vi "McP Calibrate.vi"(0 "File Info In":T2={"FilePath"=path "/DATA/Labview Items", "Field (T)"=12.0, "Temperature (K)"=12.0, "X-Axis"=enum."nm", "Center nm"=-1.0, "Current Grating Density"=enum."600", "CCD Parameters"={"Exposure Time (s)"=0.2, "Offset"=0.0, "BkgrdCrct"=FALSE, "Shutter"=FALSE, "Mode"=enum."Regular", "Repetition"=4, "dt or s"=0.0}, "Operation Mode"=enum."NML Data Acquisition", "Exp Index"=3, "Index_repetition"=0, "Index"=0, "Current Detector"=enum."CCD-1024x256"} {"CCD Parameters"."dt or s" format="%#.6f"; "CCD Parameters"."Repetition" min=1; "CCD Parameters"."Offset" format="%#.2f"; "CCD Parameters"."Exposure Time (s)" min=0.02 max=6000.0 format="%#.2f"; "Center nm" format="%.2f"; "Temperature (K)" format="%.2f"; "Field (T)" format="%.2f"}, 11 "error in":errorcluster) -> (15 "error out":errorcluster)   [LabVIEW 2024]
doc: "If you enter this program by mistake, click RETURN to quit.\n\nCALIBRATION STEPS:\n\n(0) Make sure you have calibration source (Ne lamp, Hg lamp, etc.) set up correctly.\n(1) Select a calibration line.\n(2) Click Calibrate.\n The spectrometer will move to the selected calibration line wavelength, take a CCD shot and fit the result.\n(3)Check the calibration result. You will be prompt whether to accept the result.\n (3a)Click \"Cancel\" to leave the system unaltered.\n (3b)If you click \"OK\", the counter position will be set to the calibrated value.\nThe spectrometer will return to the original internal (stepper) position afterward."
uses:
  Globals and TypeDefs/Type Definitions.llb/FileInfoParameter.ctt
  Globals and TypeDefs/Type Definitions.llb/Wavelength Unit.ctt
  Globals and TypeDefs/Type Definitions.llb/McPherson Grating Density.ctl
  Globals and TypeDefs/Type Definitions.llb/CCDParameter.ctt
  Globals and TypeDefs/Type Definitions.llb/OperationMode.ctt
  Globals and TypeDefs/Type Definitions.llb/ListOfDetectors.ctt
  MCP/Calibration/GlobalCalLampInfo.vi
  Globals and TypeDefs/gSpectrometer.vi
  File and save/X-Axis_Generator_morph.vi
panel:
  in  "Rejecting":bool
  in  "Accepting":bool
  out "Standard Wavelengths":cluster{"Y":dbl[], "Y":dbl[]}[](graph)=[{"Y"=[302.70159912109375, 302.88641357421875, 319.8586120605469, 332.37451171875, 337.82159423828125, 352.047119140625, 376.6258850097656, 377.7132873535156, 540.05615234375, 585.248779296875, 602.9996948242188, 607.4337768554688, 614.3062744140625, 616.359375, 621.7281494140625, 626.6494750976562, 638.2991943359375, 640.2247924804688, 650.65283203125, 659.895263671875, 692.9467163085938, 703.2413330078125, 717.393798828125, 724.5166625976562, 837.7608032226562, 865.4382934570312, 878.062255859375, 878.3753051757812, 1114.302001953125, 1117.75244140625, 1152.2745361328125], "Y"=[300.0, 300.0, 500.0, 1000.0, 500.0, 100.0, 800.0, 1000.0, 200.0, 200.0, 100.0, 100.0, 100.0, 100.0, 100.0, 100.0, 100.0, 200.0, 150.0, 100.0, 1000.0, 800.0, 800.0, 800.0, 800.0, 600.0, 600.0, 400.0, 300.0, 500.0, 300.0]}, {"Y"=[205.28280639648438, 226.22230529785156, 253.65170288085938, 284.7674865722656, 296.7279968261719, 365.0152893066406, 398.3930969238281, 404.65631103515625, 435.8327941894531, 542.5253295898438, 546.073486328125, 567.7105102539062, 614.947509765625, 794.4555053710938, 1013.9760131835938], "Y"=[400.0, 400.0, 1000.0, 400.0, 250.0, 600.0, 1000.0, 400.0, 1000.0, 80.0, 500.0, 200.0, 250.0, 250.0, 200.0]}, {"Y"=[427.7528076171875, 434.806396484375, 460.9566955566406, 472.6867980957031, 476.48651123046875, 480.60198974609375, 487.98638916015625, 696.5430908203125, 706.7218017578125, 750.3869018554688, 763.5106201171875, 794.817626953125, 800.61572265625, 801.4785766601562, 810.3693237304688, 811.5311279296875, 912.2966918945312, 965.7786254882812], "Y"=[200.0, 250.0, 200.0, 200.0, 250.0, 200.0, 250.0, 300.0, 300.0, 600.0, 700.0, 600.0, 600.0, 700.0, 600.0, 1000.0, 1000.0, 700.0]}]
  in  "Range":T1={"X_Min"=0.3, "X_Max"=0.3, "Y_Min"=0.3, "Y-Max"=0.3}
  out "Solved Central WL":dbl=517.6607981427933 format="%.4f"
  in  "Searching center":dbl format="%.2f"
  in  "Recalculate":bool
  out "Pre-Cal WL":dbl=6000.0 min=0.0 max=26000.0 format="%.2f"
  out "Calibration State":T8(ring)
  in  "Return?":bool
  out "cursor position":dbl format="%.4f"
  in  "Points Between":i32=10 min=0 step=1
  out "Difference (cm-1)":dbl caption="(cm-1)" format="%#_3g"
  out "Difference (meV)":dbl caption="(meV)" format="%#_3g"
  out "Difference":dbl caption="(nm)" format="%#_3g"
  out "Calibrated Wavelenth(nm)":dbl=1000.0 format="%.4f"
  out "peak plot (post-cal":cluster{"X-axis":dbl[], dbl[]}[](graph)
  out "Full Data Plot":cluster{"X-axis":dbl[], "The Data":dbl[]}(graph)
  in  "Exposuretime (s)":dbl=0.5 format="%.2f"
  out "Pre & Current WL":dbl=692.9467 caption="PreCalibrated Wavelength (nm)" format="%.4f"
  in  "Select WL":u16(ring)=5 caption="Select a Calibration Line" items=["808.2458  nm  ( Ne )", "794.3181  nm  ( Ne )", "743.8898  nm  ( Ne )", "724.5167  nm  ( Ne )", "717.3938  nm  ( Ne )", "703.2413  nm  ( Ne )", "692.9467  nm  ( Ne )", "671.7043  nm  ( Ne )", "667.8276  nm  ( Ne )", "659.8953  nm  ( Ne )", "653.2882  nm  ( Ne )", "650.6528  nm  ( Ne )", "640.2246  nm  ( Ne )", "638.2991  nm  ( Ne )", "633.4428  nm  ( Ne )", "632.8165  nm  ( Ne )", "579.2200  nm  ( Hg )", "577.1100  nm  ( Hg )", "546.2200  nm  ( Hg )", "435.9500  nm  ( Hg )", "407.8900  nm  ( Hg )", "404.7700  nm  ( Hg )", "366.4300  nm  ( Hg )", "365.5900  nm  ( Hg )", "365.1200  nm  ( Hg )", "Input Wavelength"]
  in  "StartCal":bool
  in  "Cal WL":dbl=692.9467 caption="Input Calibration Wavelength (nm)" format="%.4f"
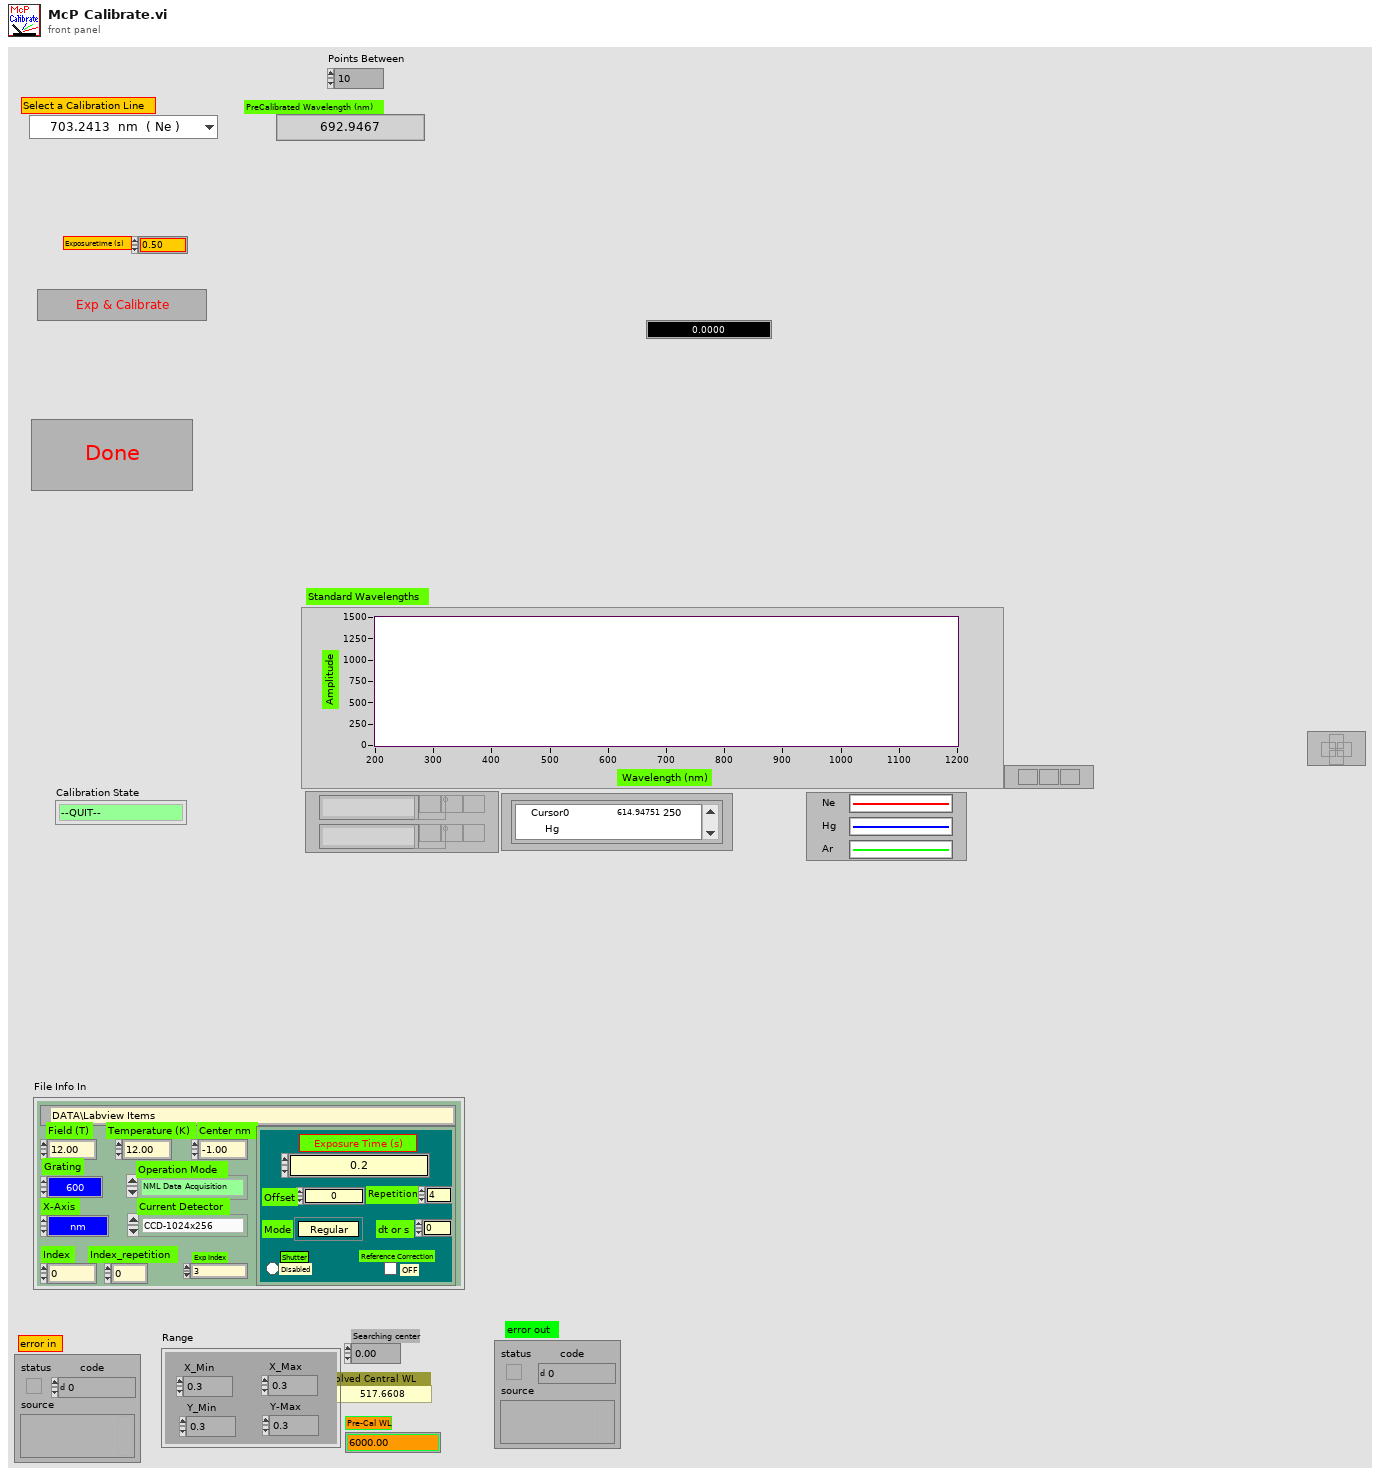
[diagram p1: front panel]
types:
  T1 = cluster{"X_Min":dbl, "X_Max":dbl, "Y_Min":dbl, "Y-Max":dbl}
  T2 = typedef "FileInfoParameter.ctt" = cluster{"FilePath":path, "Field (T)":dbl, "Temperature (K)":dbl, "X-Axis":T3, "Center nm":dbl, "Current Grating Density":T4, "CCD Parameters":T5, "Operation Mode":T6, "Exp Index":u32, "Index_repetition":u16, "Index":u16, "Current Detector":T7}
  T3 = typedef "Wavelength Unit.ctt" = enum8{"Point", "nm", "eV", "meV", "cm_1"}
  T4 = typedef "McPherson Grating Density.ctl" = enum8{"150", "300", "600", "1200", "1800"}
  T5 = typedef "CCDParameter.ctt" = cluster{"Exposure Time (s)":dbl, "Offset":dbl, "BkgrdCrct":bool, "Shutter":bool, "Mode":enum8{"Regular", "OverExp Cor", "SpikeRemove", "ForCalibration"}, "Repetition":u16, "dt or s":dbl}
  T6 = typedef "OperationMode.ctt" = enum16{"Standby", "CCD Single Shot", "CCD Sequence Shots", "CCD Custom Shots", "CCD Reference Shot", "Step Scanning ", "Time Scanning", "NML Data Acquisition"}
  T7 = typedef "ListOfDetectors.ctt" = enum8{"CCD-1024x256", "InGaAs PDA-1024x1", "CCD-1340x400", "Ge Single Channel", "Si Single Channel", "PMT Single Channel"}
  T8 = enum16{"--QUIT--", "Init", "Error", "Cancel", "Standby", "MoveToCalWL_and_Exposure", "Calculation", "Accepting the result?"}
  T9 = enum16{"Linear", "Polynomial", "Spline", "Rational"}
  T10 = cluster{"Element":string, "Wavelength":dbl, "CalWidth":dbl}[]
  T11 = cluster{"Element":string, "Wavelength":dbl, "CalWidth":dbl}
  T12 = cluster{"Post-Cal X-Axis":dbl[], "Interpolated Data":dbl[]}
  T13 = cluster{"Post-Cal X-Axis":dbl[], "Peak Amplitudes":dbl[]}
  T14 = cluster{"X-axis  (nm)":dbl[], "The Data":dbl[]}[]
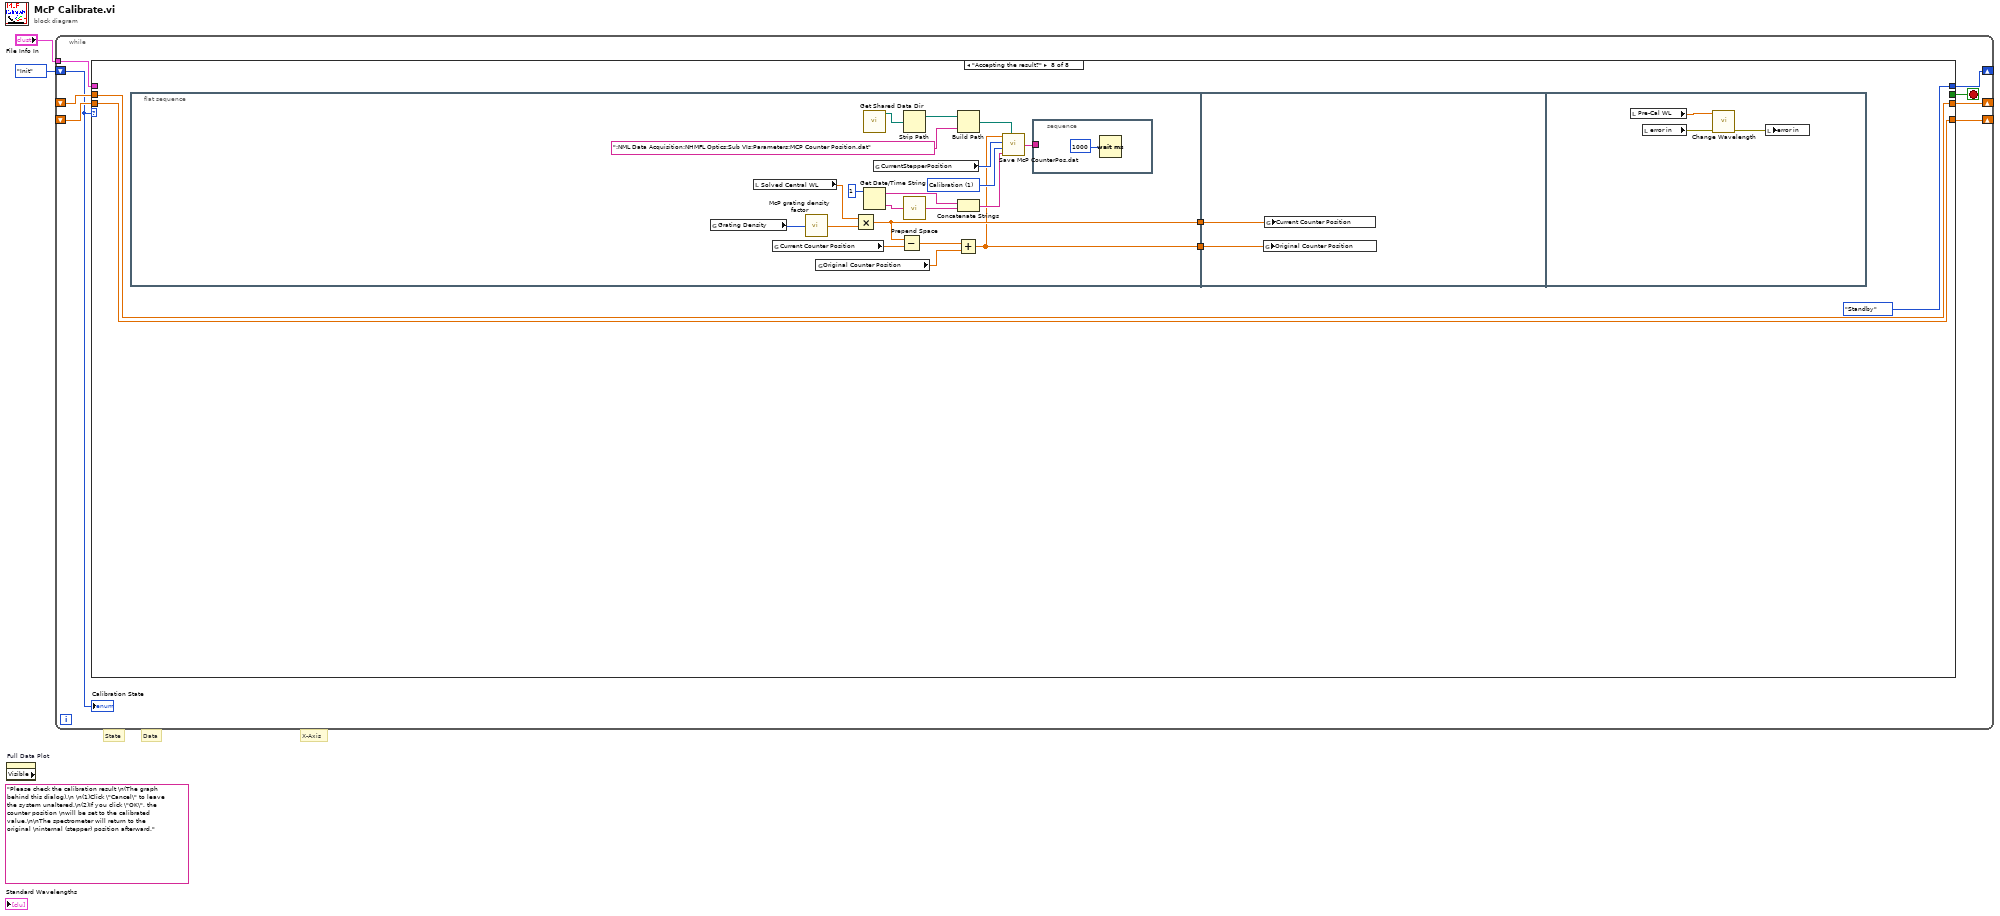
[diagram p0: block diagram]
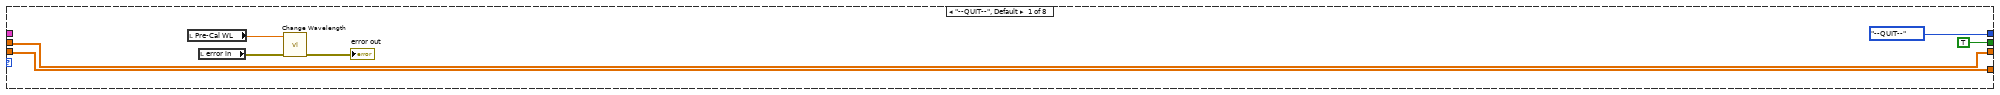
[diagram p2: hidden frame]
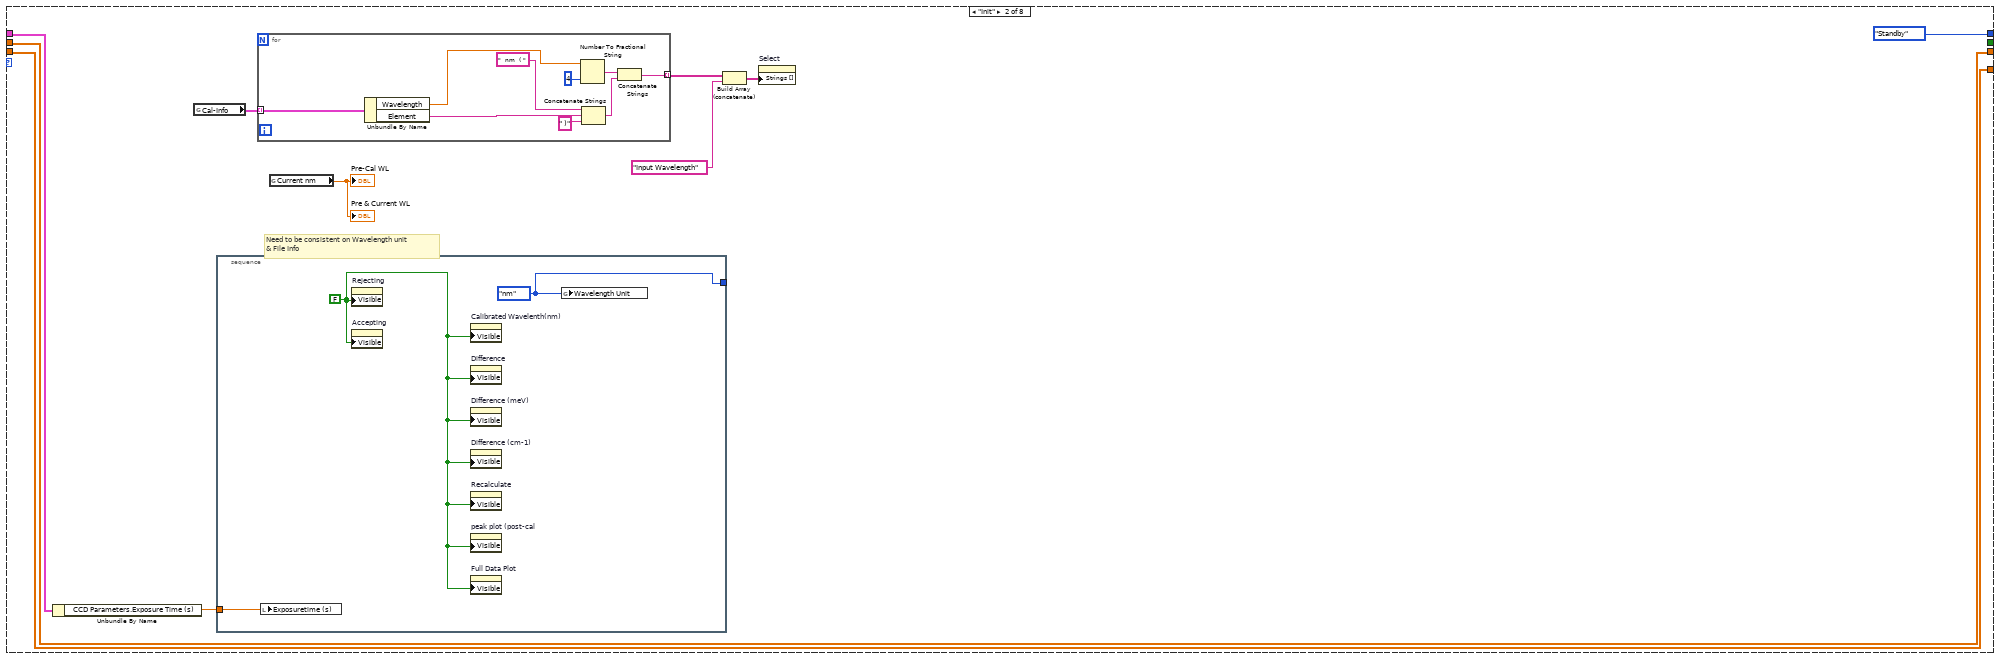
[diagram p3: hidden frame]
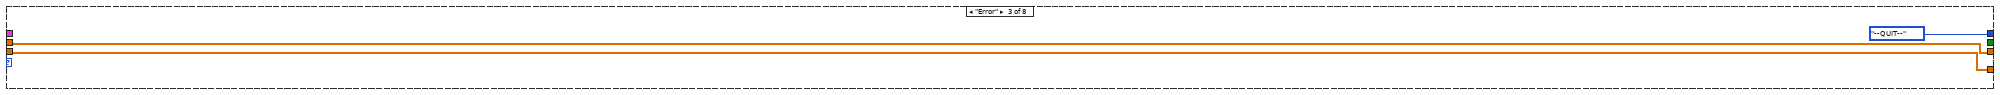
[diagram p4: hidden frame]
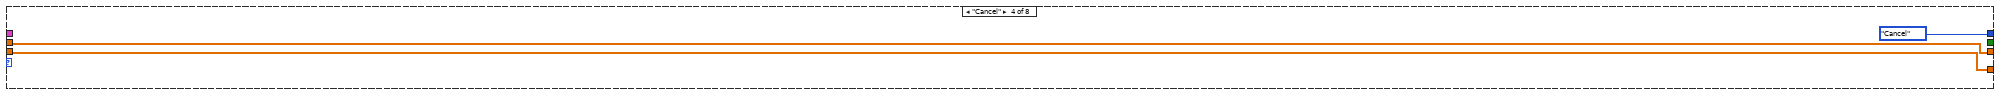
[diagram p5: hidden frame]
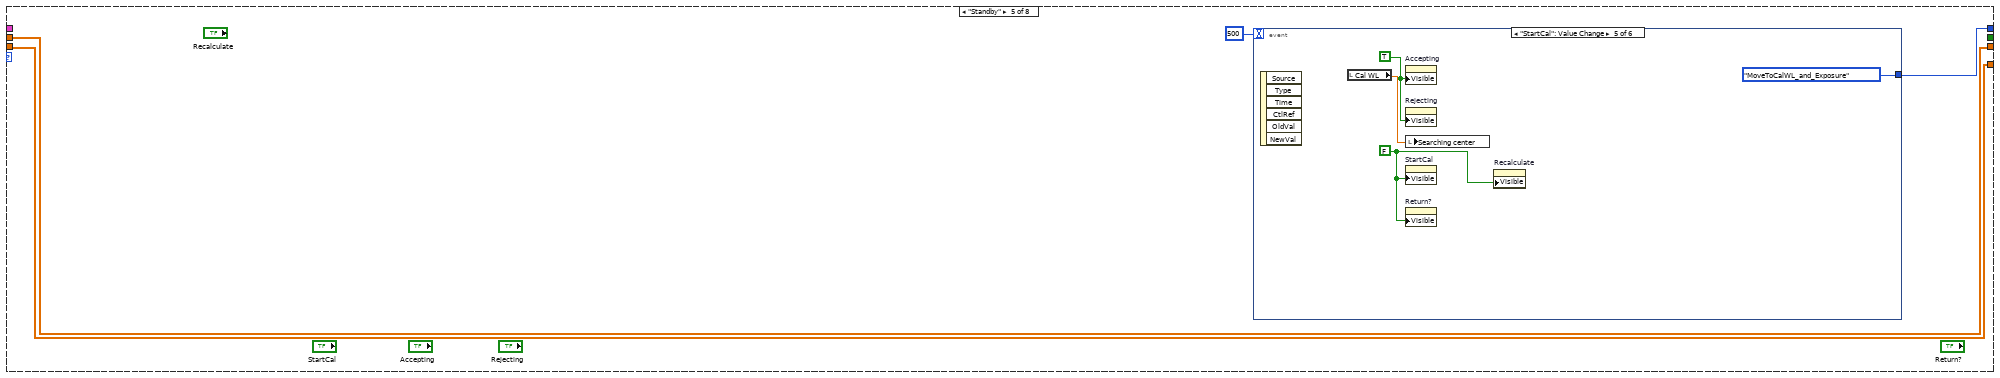
[diagram p6: hidden frame]
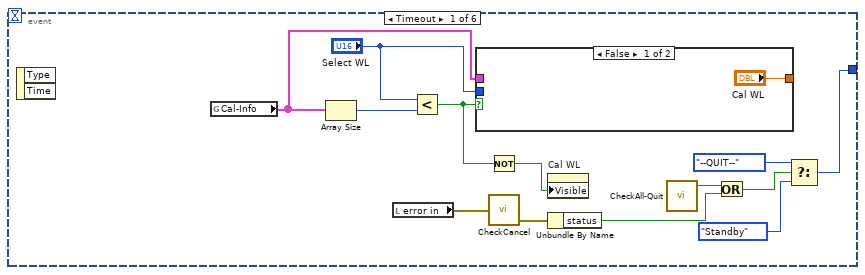
[diagram p7: hidden frame]
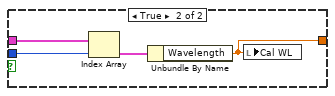
[diagram p8: hidden frame]
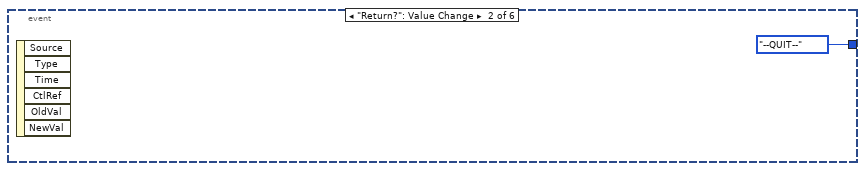
[diagram p9: hidden frame]
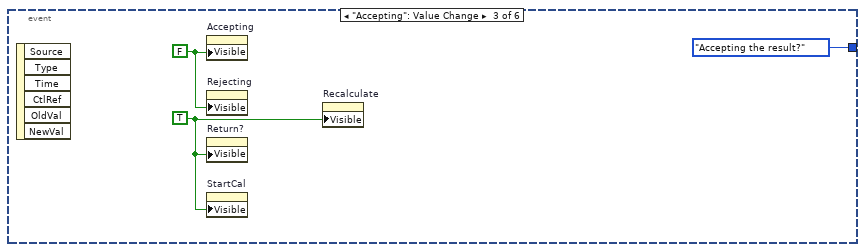
[diagram p10: hidden frame]
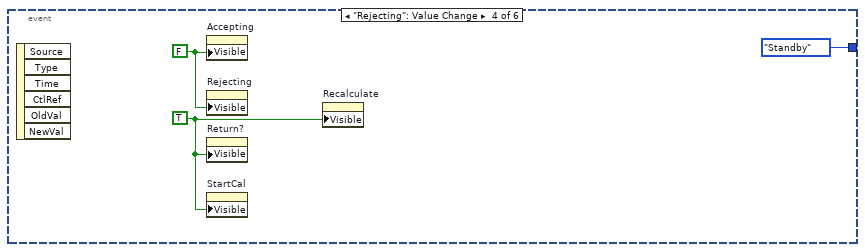
[diagram p11: hidden frame]
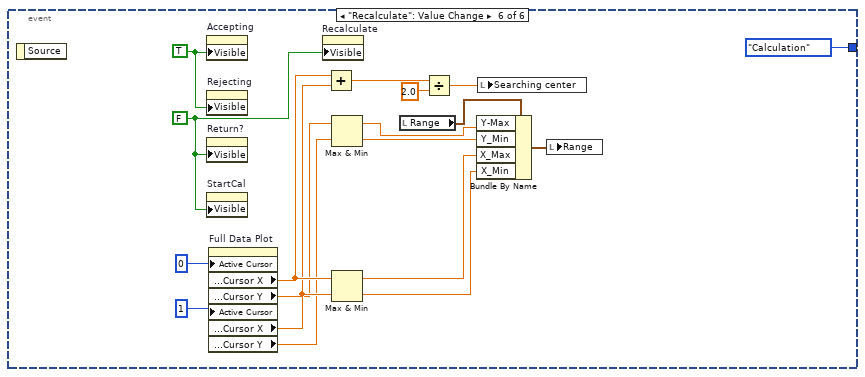
[diagram p12: hidden frame]
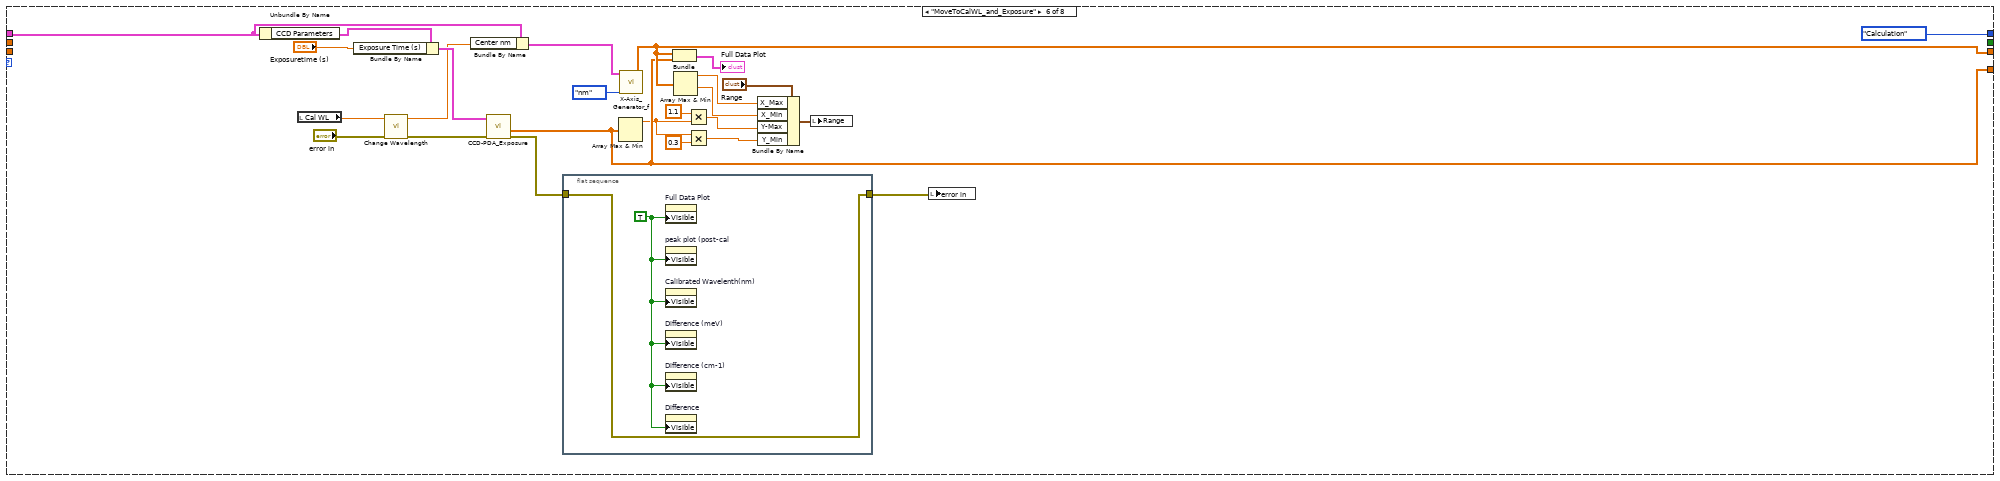
[diagram p13: hidden frame]
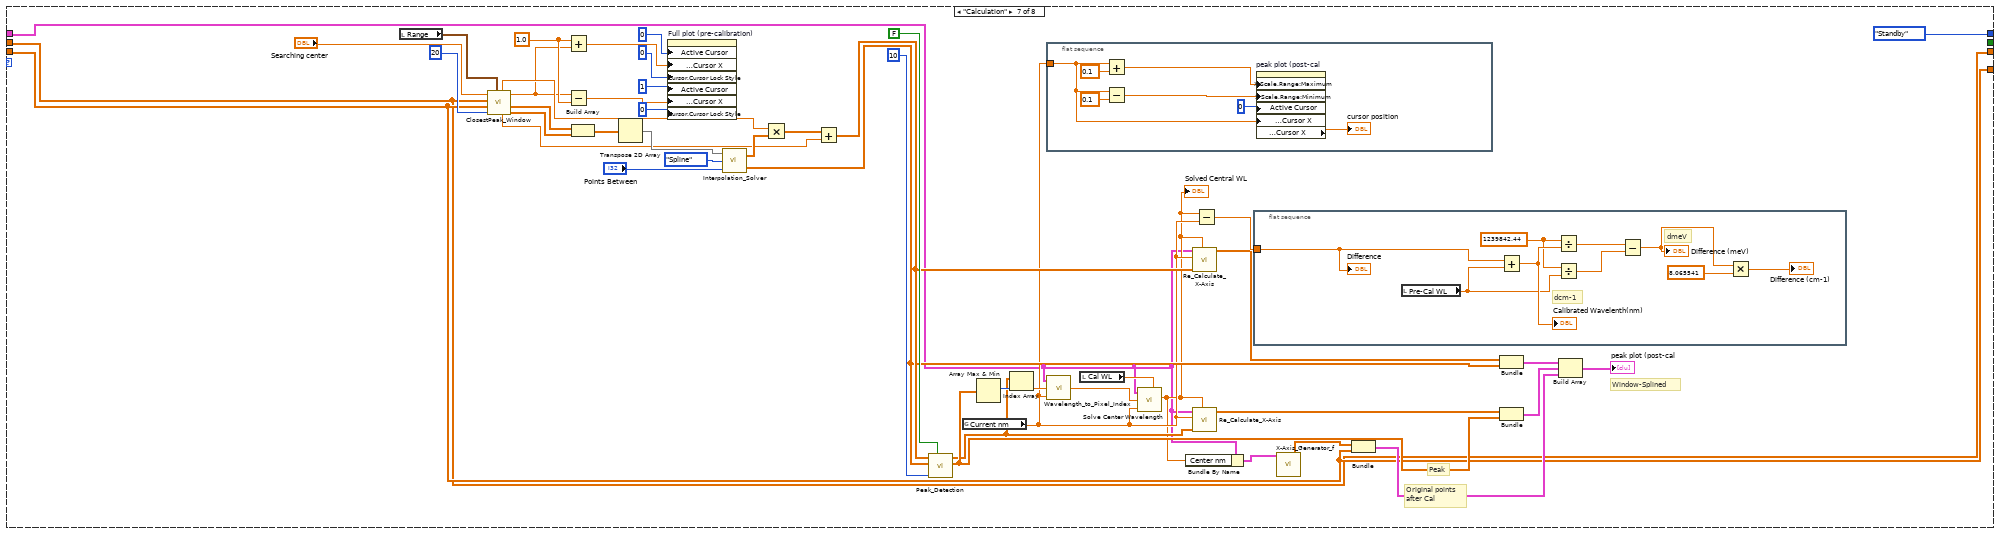
[diagram p14: hidden frame]
diagram:
  (unwired) "Please check the calibration result \n(The graph behind this dialog).\n \n(1)Click \"Cancel\" to leave the system unaltered.\n(2)If you click \"OK\", the counter position \nwill be set to the calibrated value.\n\nThe spectrometer will return to the original \ninternal (stepper) position afterward." ("message")
  # "Data"
  # "X-Axis"
  # "State"
  n1 = property on="Full Data Plot" class="XYGraph (strict)" props=["Visible"]() -> ()  [unwired: 2 in, 3 out]
  n2 = while {
    shift-right: [w10] -> _
    shift-left: _ -> [w8]
    shift-right: [w9] -> _
    shift-left: _ -> [w7]
    shift-right: [w5] -> _
    shift-left: T8."Init" ("Calibration State") -> [w3]
    tunnel: "File Info In" -> [w6]
    stop <- w4 stop-if-true
    n3 = case shown="\"Accepting the result?\"" w3 {
      tunnel: [w17 w20 w42 w45 w48 w112 w128 w190] -> w10
      tunnel: [w16 w19 w41 w44 w47 w109 w129 w189] -> w9
      tunnel: w8 -> [w17 w20 w42 w45 w48 _ w128 w190]
      tunnel: w7 -> [w16 w19 w41 w44 w47 _ w129 w189]
      tunnel: w6 -> [_ w18 _ _ _ w101 w125 _]
      tunnel: [T8."--QUIT--" ("Calibration State") T8."Standby" ("Calibration State") T8."--QUIT--" ("Calibration State") T8."Cancel" ("Calibration State") w46 T8."Calculation" ("Calibration State") T8."Standby" ("Calibration State") T8."Standby" ("Calibration State")] -> w5
      tunnel: [TRUE _ _ _ _ _ _ _] -> w4
      frame "--QUIT--", Default {
        n4 = local read "Pre-Cal WL"() -> (w13:dbl)
        n5 = local read "error in"() -> (w11:errorcluster)
        n6 = call "Change Wavelength.vi"("error in"=w11, "GOTO"=w13) -> ("error out"=→"error out":errorcluster)  [unwired: 6 in, 2 out]
      }
      frame "Init" {
        # "Need to be consistent on Wavelength unit\n& File Info"
        n7 = Unbundle By Name(w18) -> ("CCD Parameters.Exposure Time (s)"=w27:dbl)
        n8 = global read "GlobalCalLampInfo.vi" "Cal-Info"() -> (w23:T10)
        n9 = stacked-sequence {
          tunnel: [w38] -> _
          tunnel: w27 -> [w39]
          frame #0 {
            w38 = Wavelength_Unit.ctt."nm" ("Wavelength Unit")
            w37 = FALSE ("Visible")
            n10 = local write "Exposuretime (s)"(w39) -> ()
            n11 = property on="Rejecting" class="Bool"("Visible"=w37) -> ()  [unwired: 2 in, 2 out]
            n12 = property on="Accepting" class="Bool"("Visible"=w37) -> ()  [unwired: 2 in, 2 out]
            n13 = property on="Calibrated Wavelenth(nm)" class="DigNum (strict)"("Visible"=w37) -> ()  [unwired: 2 in, 2 out]
            n14 = property on="Difference" class="DigNum (strict)"("Visible"=w37) -> ()  [unwired: 2 in, 2 out]
            n15 = property on="Difference (meV)" class="DigNum (strict)"("Visible"=w37) -> ()  [unwired: 2 in, 2 out]
            n16 = property on="Difference (cm-1)" class="DigNum (strict)"("Visible"=w37) -> ()  [unwired: 2 in, 2 out]
            n17 = property on="Recalculate" class="Bool"("Visible"=w37) -> ()  [unwired: 2 in, 2 out]
            n18 = property on="peak plot (post-cal" class="XYGraph (strict)"("Visible"=w37) -> ()  [unwired: 2 in, 2 out]
            n19 = property on="Full Data Plot" class="XYGraph (strict)"("Visible"=w37) -> ()  [unwired: 2 in, 2 out]
            n20 = global write "gSpectrometer.vi" "Wavelength Unit"(w38) -> ()
          }
        }
        n21 = for {
          tunnel: w23 -> [w36] mode=indexing
          tunnel: [w34] -> w24 mode=indexing
          n22 = Unbundle By Name(w36) -> ("Wavelength"=w33:dbl, "Element"=w30:string)
          n23 = Number To Fractional String(number=w33, precision (6)=4) -> (F-format string=w32:string)  [unwired: 2 in]
          n24 = Concatenate Strings("  nm  ( ", w30, " )") -> (w28:string)
          n25 = Concatenate Strings(w32, w28) -> (w34:string)
        }
        n26 = global read "gSpectrometer.vi" "Current nm"() -> (→"Pre & Current WL" →"Pre-Cal WL":dbl)
        n27 = Build Array (concatenate)(w24, "Input Wavelength") -> (w26:string[])
        n28 = property on="Select" class="Ring (strict)"("Strings []"=w26) -> ()  [unwired: 2 in, 2 out]
      }
      frame "Error" {
      }
      frame "Cancel" {
      }
      frame "Standby" {
        n29 = event shown="[4] \"StartCal\": Value Change" {
          selector: _ -> [_ _ _ _ _ _]
          dyn-events: _ -> [_ _ _ _ _ _]
          timeout: 500 -> [_ _ _ _ _ _]
          tunnel: [w54 T8."--QUIT--" ("Calibration State") T8."Accepting the result?" ("Calibration State") T8."Standby" ("Calibration State") T8."MoveToCalWL_and_Exposure" ("Calibration State") T8."Calculation" ("Calibration State")] -> w46
          event Timeout {
            n30 = event-data() -> ()  [unwired: 1 in, 2 out]
            n31 = global read "GlobalCalLampInfo.vi" "Cal-Info"() -> (w58:T10)
            n32 = Array Size(array=w58) -> (size(s)=w62:i32)
            n33 = local read "error in"() -> (w52:errorcluster)
            n34 = Less?(x="Select WL", y=w62) -> (x < y?=w59:bool)
            n35 = case shown="False" w59 {
              tunnel: ["Cal WL" w65] -> _
              tunnel: w58 -> [_ w66]
              tunnel: "Select WL" -> [_ w64]
              frame False {
              }
              frame True {
                n36 = Index Array(array=w66, index=w64) -> (element=w67:T11)
                n37 = Unbundle By Name(w67) -> ("Wavelength"=w65:dbl)
                n38 = local write "Cal WL"(w65) -> ()
              }
            }
            n39 = Not(x=w59) -> (.not. x?=w60:bool)
            n40 = call "CheckCancel.vi"("error in (no error)"=w52) -> ("error out"=w51:errorcluster)  [unwired: 1 in, 1 out]
            n41 = property on="Cal WL" class="DigNum (strict)"("Visible"=w60) -> ()  [unwired: 2 in, 2 out]
            n42 = Unbundle By Name(w51) -> ("status"=w50:bool)
            n43 = call "CheckAll-Quit.vi"() -> ("All-Quit"=w57:bool)  [unwired: 3 in]
            n44 = Or(x=w57, y=w50) -> (x .or. y?=w56:bool)
            n45 = Select(t=T8."--QUIT--", s=w56, f=T8."Standby" ("Calibration State")) -> (s? t:f=w54:T8)
          }
          event "Return?": Value Change {
            n46 = event-data() -> ()  [unwired: 1 in, 6 out]
          }
          event "Accepting": Value Change {
            w70 = TRUE ("Visible")
            w69 = FALSE ("Visible")
            n47 = event-data() -> ()  [unwired: 1 in, 6 out]
            n48 = property on="Accepting" class="Bool"("Visible"=w69) -> ()  [unwired: 2 in, 2 out]
            n49 = property on="Rejecting" class="Bool"("Visible"=w69) -> ()  [unwired: 2 in, 2 out]
            n50 = property on="Return?" class="Bool"("Visible"=w70) -> ()  [unwired: 2 in, 2 out]
            n51 = property on="StartCal" class="Bool"("Visible"=w70) -> ()  [unwired: 2 in, 2 out]
            n52 = property on="Recalculate" class="Bool"("Visible"=w70) -> ()  [unwired: 2 in, 2 out]
          }
          event "Rejecting": Value Change {
            w72 = TRUE ("Visible")
            w73 = FALSE ("Visible")
            n53 = event-data() -> ()  [unwired: 1 in, 6 out]
            n54 = property on="Accepting" class="Bool"("Visible"=w73) -> ()  [unwired: 2 in, 2 out]
            n55 = property on="Rejecting" class="Bool"("Visible"=w73) -> ()  [unwired: 2 in, 2 out]
            n56 = property on="Return?" class="Bool"("Visible"=w72) -> ()  [unwired: 2 in, 2 out]
            n57 = property on="StartCal" class="Bool"("Visible"=w72) -> ()  [unwired: 2 in, 2 out]
            n58 = property on="Recalculate" class="Bool"("Visible"=w72) -> ()  [unwired: 2 in, 2 out]
          }
          event "StartCal": Value Change {
            w75 = TRUE ("Visible")
            w76 = FALSE ("Visible")
            n59 = event-data() -> ()  [unwired: 1 in, 6 out]
            n60 = local read "Cal WL"() -> (w78:dbl)
            n61 = property on="Accepting" class="Bool"("Visible"=w75) -> ()  [unwired: 2 in, 2 out]
            n62 = property on="Rejecting" class="Bool"("Visible"=w75) -> ()  [unwired: 2 in, 2 out]
            n63 = property on="StartCal" class="Bool"("Visible"=w76) -> ()  [unwired: 2 in, 2 out]
            n64 = property on="Return?" class="Bool"("Visible"=w76) -> ()  [unwired: 2 in, 2 out]
            n65 = local write "Searching center"(w78) -> ()
            n66 = property on="Recalculate" class="Bool"("Visible"=w76) -> ()  [unwired: 2 in, 2 out]
          }
          event "Recalculate": Value Change {
            w79 = TRUE ("Visible")
            w80 = FALSE ("Visible")
            n67 = event-data() -> ()  [unwired: 1 in, 1 out]
            n68 = property on="Accepting" class="Bool"("Visible"=w79) -> ()  [unwired: 2 in, 2 out]
            n69 = property on="Rejecting" class="Bool"("Visible"=w79) -> ()  [unwired: 2 in, 2 out]
            n70 = property on="Return?" class="Bool"("Visible"=w80) -> ()  [unwired: 2 in, 2 out]
            n71 = property on="StartCal" class="Bool"("Visible"=w80) -> ()  [unwired: 2 in, 2 out]
            n72 = property on="Full Data Plot" class="XYGraph (strict)"("Active Cursor"=u32 0, "Active Cursor"=u32 1) -> ("Cursor.Cursor Position:Cursor X"=w90:dbl, "Cursor.Cursor Position:Cursor Y"=w88:dbl, "Cursor.Cursor Position:Cursor X"=w89:dbl, "Cursor.Cursor Position:Cursor Y"=w87:dbl)  [unwired: 2 in, 2 out]
            n73 = property on="Recalculate" class="Bool"("Visible"=w80) -> ()  [unwired: 2 in, 2 out]
            n74 = Add(x=w90, y=w89) -> (x+y=w94:dbl)
            n75 = Max & Min(x=w88, y=w87) -> (max(x,y)=w85:dbl, min(x,y)=w84:dbl)
            n76 = Max & Min(x=w90, y=w89) -> (max(x,y)=w83:dbl, min(x,y)=w82:dbl)
            n77 = local read "Range"() -> (w86:T1)
            n78 = Divide(x=w94, y=2.0) -> (x/y=w92:dbl)
            n79 = Bundle By Name(cluster=w86, "Y-Max"=w85, "Y_Min"=w84, "X_Max"=w83, "X_Min"=w82) -> (w81:T1)
            n80 = local write "Searching center"(w92) -> ()
            n81 = local write "Range"(w81) -> ()
          }
        }
      }
      frame "MoveToCalWL_and_Exposure" {
        n82 = Unbundle By Name(w101) -> ("CCD Parameters"=w114:T5)
        n83 = local read "Cal WL"() -> (w116:dbl)
        n84 = Bundle By Name(cluster=w114, "Exposure Time (s)"="Exposuretime (s)") -> (w117:T5)
        n85 = call "Change Wavelength.vi"("error in"="error in", "GOTO"=w116) -> ("error out"=w118:errorcluster, "Final nm"=w97:dbl)  [unwired: 6 in, 1 out]
        n86 = Bundle By Name(cluster=w101, "Center nm"=w97) -> (w100:T2)
        n87 = call "CCD-PDA_Exposure.vi"("error in"=w118, "CCD Parameters"=w117) -> ("Error Out"=w99:errorcluster, "The Data"=w109:dbl[])  [unwired: 3 in, 2 out]
        n88 = flat-sequence {
          tunnel: w99 -> [w123]
          tunnel: [w123] -> w98
          frame #0 {
            w122 = TRUE
            n89 = property on="Full Data Plot" class="XYGraph (strict)"("Visible"=w122) -> ()  [unwired: 2 in, 2 out]
            n90 = property on="peak plot (post-cal" class="XYGraph (strict)"("Visible"=w122) -> ()  [unwired: 2 in, 2 out]
            n91 = property on="Calibrated Wavelenth(nm)" class="DigNum (strict)"("Visible"=w122) -> ()  [unwired: 2 in, 2 out]
            n92 = property on="Difference (meV)" class="DigNum (strict)"("Visible"=w122) -> ()  [unwired: 2 in, 2 out]
            n93 = property on="Difference (cm-1)" class="DigNum (strict)"("Visible"=w122) -> ()  [unwired: 2 in, 2 out]
            n94 = property on="Difference" class="DigNum (strict)"("Visible"=w122) -> ()  [unwired: 2 in, 2 out]
          }
        }
        n95 = Array Max & Min(array=w109) -> (max value=w104:dbl)  [unwired: 3 out]
        n96 = call-poly "X-Axis_Generator_f.vi"("File Info In"=w100, "X-Axis Unit"=Wavelength_Unit.ctt."nm") -> ("X-axis  (nm)"=w112:dbl[])  [unwired: 10 in, 7 out]
        n97 = Bundle("X-axis  (nm)"=w112, "The Data"=w109) -> (→"Full Data Plot":cluster{"X-axis  (nm)":dbl[], "The Data":dbl[]})  [unwired: 1 in]
        n98 = Array Max & Min(array=w112) -> (max value=w111:dbl, min value=w110:dbl)  [unwired: 2 out]
        n99 = Multiply(x=1.1, y=w104) -> (x*y=w103:dbl)
        n100 = Multiply(x=w104, y=0.3) -> (x*y=w107:dbl)
        n101 = Bundle By Name(cluster="Range", "X_Max"=w111, "X_Min"=w110, "Y-Max"=w103, "Y_Min"=w107) -> (w106:T1)
        n102 = local write "Range"(w106) -> ()
        n103 = local write "error in"(w98) -> ()
      }
      frame "Calculation" {
        w141 = 1.0
        # "Original points\nafter Cal"
        # "Peak"
        # "Window-Splined"
        n104 = local read "Range"() -> (w127:T1)
        n105 = call "ClosestPeak_Window.vi"("Range"=w127, "Window Width (point)"=20, "The Data"=w129, "X-axis"=w128, "Searching center"="Searching center") -> ("Data Subset"=w167:dbl[], "X-Axis Subset"=w166:dbl[], "Closest peak position"=w132:dbl, "starting point"=w160:dbl, "scale"=w159:dbl)  [unwired: 2 in]
        n106 = Add(x=w141, y=w132) -> (x+y=w136:dbl)
        n107 = Subtract(x=w132, y=w141) -> (x-y=w135:dbl)
        n108 = Build Array(w166, w167) -> (w164:dbl[][])
        n109 = Transpose 2D Array(2D array=w164) -> (transposed array=w165:dbl[][])
        n110 = property on="Full plot (pre-calibration)" class="XYGraph (strict)"("Active Cursor"=u32 0, "Cursor.Cursor Position:Cursor X"=w136, "Cursor.Cursor Lock Style"=u32 0 ("Cursor Locked"), "Active Cursor"=u32 1, "Cursor.Cursor Position:Cursor X"=w135, "Cursor.Cursor Lock Style"=u32 0 ("Cursor Locked")) -> ()  [unwired: 2 in, 2 out]
        n111 = call "Interpolation_Solver.vi"("Points Between"="Points Between", "Type of Interpolation"=T9."Spline", "Data"=w165) -> ("Interpolated Data"=w146:dbl[], "Interpolated X Axis"=w168:dbl[])
        n112 = Multiply(x=w159, y=w168) -> (x*y=w161:dbl[])
        n113 = Add(x=w161, y=w160) -> (x+y=w147:dbl[])
        n114 = call "Peak_Detection.vi"("View Result?"=FALSE, "PD width"=10 ("Points Between"), "Input y data"=w146, "Input x data"=w147) -> ("Peak Amplitudes"=w145:dbl[], "Peak Locations"=w143:dbl[])  [unwired: 1 in, 5 out]
        n115 = global read "gSpectrometer.vi" "Current nm"() -> (w131:dbl)
        n116 = Array Max & Min(array=w145) -> (max index (indices)=w153:i32)  [unwired: 3 out]
        n117 = Index Array(array=w143, index=w153) -> (element=w154:dbl)
        n118 = flat-sequence {
          tunnel: w131 -> [w170]
          frame #0 {
            n119 = Add(x=w170, y=0.1) -> (x+y=w173:dbl)
            n120 = Subtract(x=w170, y=0.1) -> (x-y=w172:dbl)
            n121 = property on="peak plot (post-cal" class="XYGraph (strict)"("X Scale.Range:Maximum"=w173, "X Scale.Range:Minimum"=w172, "Active Cursor"=u32 0, "Cursor.Cursor Position:Cursor X"=w170) -> ("Cursor.Cursor Position:Cursor X"=→"cursor position":dbl)  [unwired: 2 in, 2 out]
          }
        }
        n122 = call "Wavelength_to_Pixel_Index.vi"("Central Wavelength"=w131, "Wavelength for Pixel i"=w154, "File Info In"=w125) -> ("index (out)"=w155:dbl)  [unwired: 2 in]
        n123 = local read "Cal WL"() -> (w134:dbl)
        n124 = call "Solve Center Wavelength.vi"("Standard Wavelength"=w134, "Current Central Wavelength"=w131, "pixel index"=w155, "File Info"=w125) -> ("Solved Central Wavelength for Calibration"=w126:dbl)  [unwired: 4 in]
        "Solved Central WL" <- w126
        n125 = Bundle By Name(cluster=w125, "Center nm"=w126) -> (w124:T2)
        n126 = call "Re_Calculate_X-Axis.vi"("Calibrated Central nm"=w126, "Pre-Cal X-Axis"=w147, "Pre-Cal Center nm"=w131, "File Info In"=w125) -> ("Post-Cal X-Axis"=w151:dbl[])  [unwired: 5 in]
        n127 = call "Re_Calculate_X-Axis.vi"("Calibrated Central nm"=w126, "Pre-Cal X-Axis"=w143, "Pre-Cal Center nm"=w131, "File Info In"=w125) -> ("Post-Cal X-Axis"=w142:dbl[])  [unwired: 5 in]
        n128 = Subtract(x=w126, y=w131) -> (x-y=w152:dbl)
        n129 = flat-sequence {
          tunnel: w152 -> [w178]
          frame #0 {
            w184 = 1239842.44
            # "dmeV"
            # "dcm-1"
            n130 = local read "Pre-Cal WL"() -> (w177:dbl)
            n131 = Add(x=w178, y=w177) -> (x+y=w185:dbl)
            "Calibrated Wavelenth(nm)" <- w185
            n132 = Divide(x=w184, y=w185) -> (x/y=w179:dbl)
            n133 = Divide(x=w184, y=w177) -> (x/y=w180:dbl)
            n134 = Subtract(x=w179, y=w180) -> (x-y=w181:dbl)
            "Difference (meV)" <- w181
            n135 = Multiply(x=w181, y=8.065541) -> (x*y=→"Difference (cm-1)":dbl)
            "Difference" <- w178
          }
        }
        n136 = call-poly "X-Axis_Generator_f.vi"("File Info In"=w124) -> ("X-axis  (nm)"=w156:dbl[])  [unwired: 11 in, 7 out]
        n137 = Bundle("X-axis  (nm)"=w156, "The Data"=w129) -> (w144:cluster{"X-axis  (nm)":dbl[], "The Data":dbl[]})  [unwired: 1 in]
        n138 = Bundle("Post-Cal X-Axis"=w151, "Interpolated Data"=w146) -> (w148:T12)  [unwired: 1 in]
        n139 = Bundle("Post-Cal X-Axis"=w142, "Peak Amplitudes"=w145) -> (w149:T13)  [unwired: 1 in]
        n140 = Build Array(w148, w149, w144) -> (→"peak plot (post-cal":T14)
      }
      frame "Accepting the result?" {
        n141 = flat-sequence {
          tunnel: [w197] -> w187
          tunnel: [w198] -> w186
          tunnel: w187 -> [w213]
          tunnel: w186 -> [w212]
          frame #0 {
            w206 = u16 1 items=["Moving", "Calibration", "Key in", "Initialization"] ("Set Method")
            n142 = global read "gSpectrometer.vi" "Grating Density"() -> (w207:T4)
            n143 = local read "Solved Central WL"() -> (w200:dbl)
            n144 = global read "gSpectrometer.vi" "Current Counter Position"() -> (w209:dbl)
            n145 = call "McP grating density factor.vi"("Grating Density"=w207) -> ("GratingFactor"=w208:dbl)
            n146 = global read "gSpectrometer.vi" "Original Counter Position"() -> (w210:dbl)
            n147 = Multiply(x=w200, y=w208) -> (x*y=w198:dbl)
            n148 = call "Get Shared Data Dir.vi"() -> ("Data Directory Path"=w192:path)  [unwired: 2 in, 1 out]
            n149 = Get Date/Time String(date format (0)=1) -> (date string=w204:string, time string=w196:string)  [unwired: 2 in]
            n150 = global read "gSpectrometer.vi" "CurrentStepperPosition"() -> (w199:i32)
            n151 = Subtract(x=w198, y=w209) -> (x-y=w202:dbl)
            n152 = Strip Path(path=w192) -> (stripped path=w193:path)  [unwired: 1 out]
            n153 = call "Prepend Space.vi"("Input String"=w196) -> ("Space + Input String"=w195:string)
            n154 = Build Path(base path=w193, name or relative path=":NML Data Acquisition:NHMFL Optics:Sub VIs:Parameters:MCP Counter Position.dat") -> (appended path=w191:path)
            n155 = Concatenate Strings(w204, w195) -> (w203:string)
            n156 = Add(x=w202, y=w210) -> (x+y=w197:dbl)
            n157 = call "Save McP CounterPos.dat.VI"("McP Counter Position Path"=w191, "Last Calibration Date"=w203, "Set Method"=w206, "McP Stepper Position"=w199, "McP Counter Position"=w197) -> ("Written content"=w201:string)  [unwired: 1 in]
            n158 = stacked-sequence {
              tunnel: w201 -> [_]
              frame #0 {
                n159 = Wait (ms)(milliseconds to wait=u32 1000) -> ()  [unwired: 1 out]
              }
            }
          }
          frame #1 {
            n160 = global write "gSpectrometer.vi" "Original Counter Position"(w213) -> ()
            n161 = global write "gSpectrometer.vi" "Current Counter Position"(w212) -> ()
          }
          frame #2 {
            n162 = local read "Pre-Cal WL"() -> (w214:dbl)
            n163 = local read "error in"() -> (w216:errorcluster)
            n164 = call "Change Wavelength.vi"("error in"=w216, "GOTO"=w214) -> ("error out"=w215:errorcluster)  [unwired: 6 in, 2 out]
            n165 = local write "error in"(w215) -> ()
          }
        }
      }
    }
    "Calibration State" <- w3
  }
